vi "Excel_CloseReference.vi"(4 "Base Path":string="C:\\Users\\TOSHIBA\\Desktop\\Excel", 5 "Visible":bool, 6 "File Name":string="denemem", 7 "Keep Excel Open ?":bool=TRUE, 8 "error in (no error)":errorcluster, 9 "Sheets Reference In":refnum<k7>, 10 "Workbook Reference In":refnum<k7>, 11 "Excel Application Reference In":refnum<k7>) -> (0 "error out":errorcluster)   [LabVIEW 2014]
doc: "This VI demonstrates the use of ActiveX to write a table into a Microsoft Excel worksheet."
panel:
  out "string":string
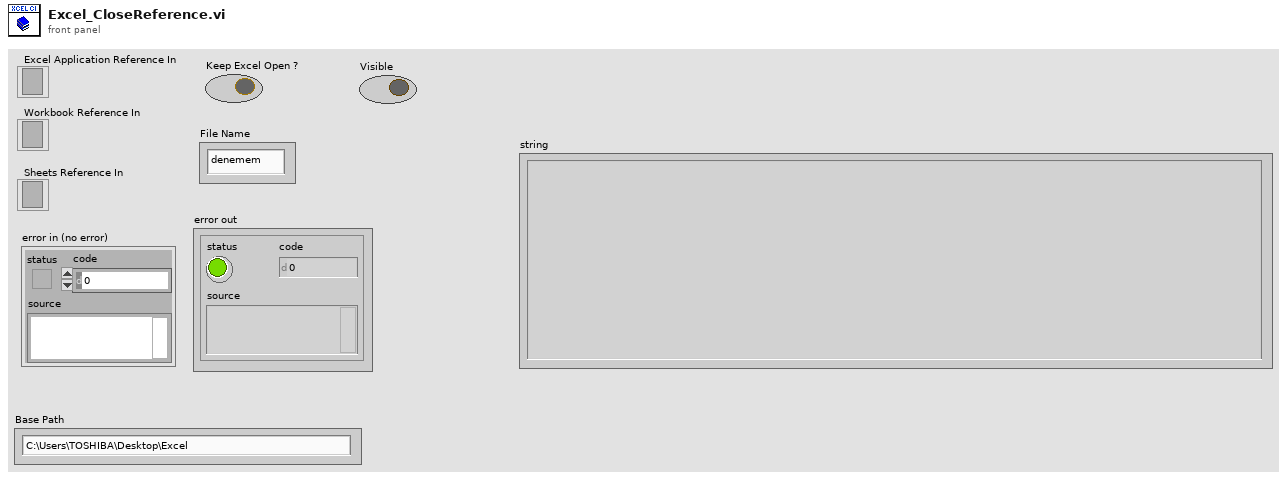
[diagram p1: front panel]
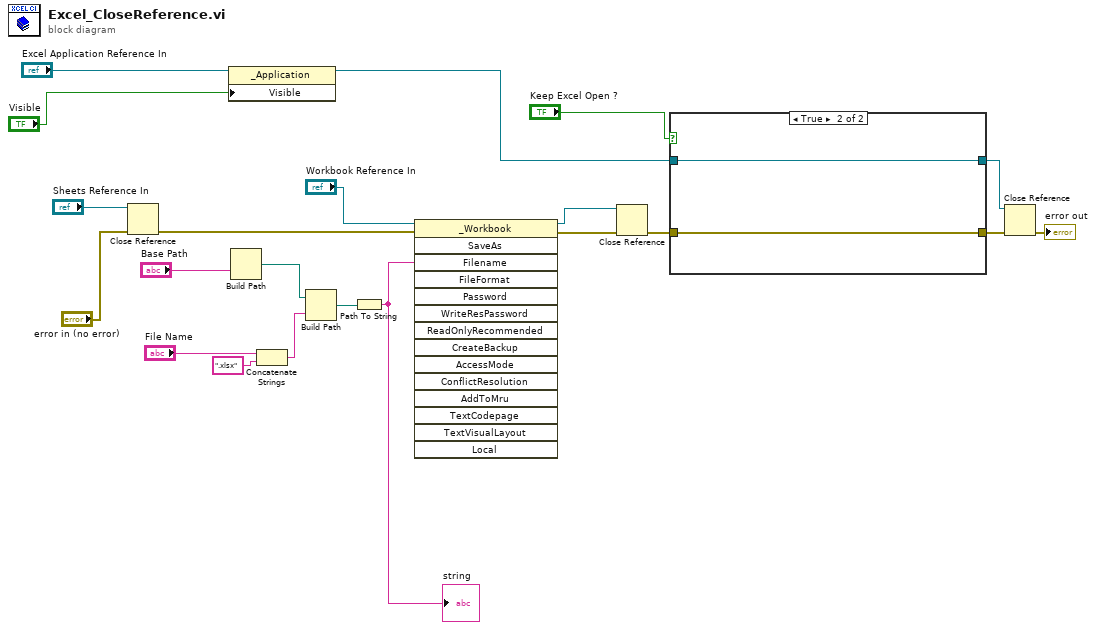
[diagram p0: block diagram]
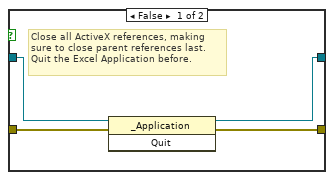
[diagram p2: hidden frame]
diagram:
  n1 = Close Reference(reference="Sheets Reference In", error in (no error)="error in (no error)") -> (error out=w3:errorcluster)
  n2 = property class="_Application"(reference="Excel Application Reference In", "Visible"="Visible") -> (reference out=w2:refnum<k7>)  [unwired: 1 in, 1 out]
  n3 = Build Path(name or relative path="Base Path") -> (appended path=w7:path)  [unwired: 1 in]
  n4 = Concatenate Strings("File Name", ".xlsx" ("string")) -> (w6:string)
  n5 = Build Path(base path=w7, name or relative path=w6) -> (appended path=w5:path)
  n6 = Path To String(path=w5) -> (string=w4:string)
  "string" <- w4
  n7 = invoke class="_Workbook" method="SaveAs"(reference="Workbook Reference In", error in=w3, "Filename"=w4) -> (reference out=w11:refnum<k7>, error out=w21:errorcluster)  [unwired: 12 in, 13 out]
  n8 = Close Reference(reference=w11, error in (no error)=w21) -> (error out=w20:errorcluster)
  n9 = case shown="True" "Keep Excel Open ?" {
    tunnel: w20 -> [w25 w26]
    tunnel: w2 -> [w24 w27]
    tunnel: [w23 w26] -> w18
    tunnel: [w22 w27] -> w17
    frame False {
      # "Close all ActiveX references, making sure to close parent references last.\nQuit the Excel Application before."
      n10 = invoke class="_Application" method="Quit"(reference=w24, error in=w25) -> (reference out=w22:refnum<k7>, error out=w23:errorcluster)  [unwired: 1 in, 1 out]
    }
    frame True {
    }
  }
  n11 = Close Reference(reference=w17, error in (no error)=w18) -> (error out=→"error out":errorcluster)
